vi "CreateEvent_Item_Init.vi"(11 "Object":T1) -> ()   [LabVIEW 2012]
doc: "Init\n\n\nInputs:\n---------------------\n- Object : U64; \n\nOutputs:\n---------------------\n\n\n----------------------------------------------\n6/8/2018 jcm\nZühlke Engineering AG\nCH-8952 Schlieren\nwww.zuehlke.com"
uses:
  <resource>/Framework/Providers/API/ItemRef.ctl
panel:
  out "error out":errorcluster
  in  "error in":errorcluster
  # "Connector Pane"
  # "Locals"
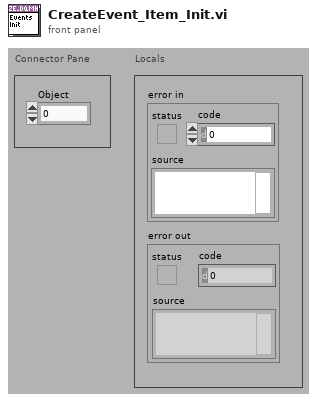
[diagram p1: front panel]
types:
  T1 = typedef "ItemRef.ctl" = u64
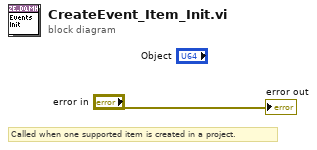
[diagram p0: block diagram]
diagram:
  # "Called when one supported item is created in a project."
  "error out" <- "error in"
